vi "emi_Error Filter Array.vi"(1 "Action(No Error)":T2, 5 "Error Codes":i32[](array[numeric]), 9 "error in (no error)":errorcluster, 12 "Filter(Error&Warning)":T1) -> (8 "Filter Triggered":bool, 10 "error out":errorcluster)   [LabVIEW 2011]
doc: "Filter error codes based on code(s). \n\nIf Code does not match, no action.\n\nIf code matches, the following is carried out:\nAction = No Error: Remove error.\nAction = Warning: Change from error to warning.\nAction = Error: Leave as Error.\nFilter Triggered is set to True.\n\nIf filtering both Warnings and errors, use bothe Error Filter.vi and Warning Filter.vi"
uses:
  emi_Error&Warning Filter Action.ctl
  _emi_Filter type.ctl
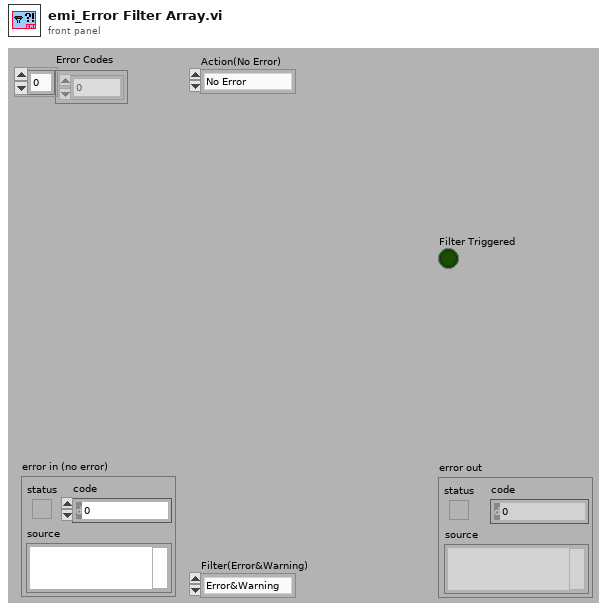
[diagram p1: front panel]
types:
  T1 = typedef "_emi_Filter type.ctl" = enum16{"Error&Warning", "Warning", "Error"}
  T2 = typedef "emi_Error&Warning Filter Action.ctl" = enum16{"No Error", "Warning", "Error"}
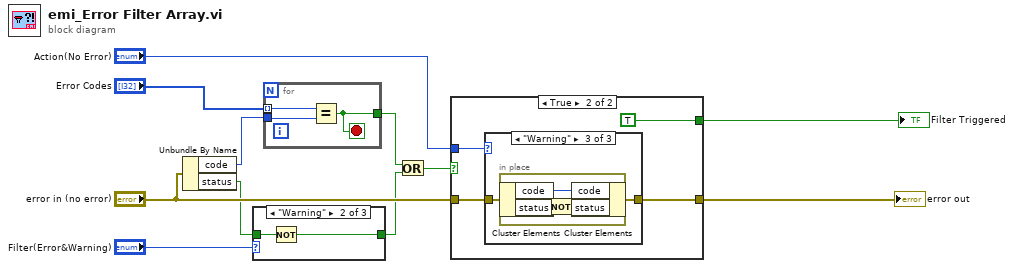
[diagram p0: block diagram]
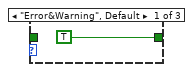
[diagram p2: hidden frame]
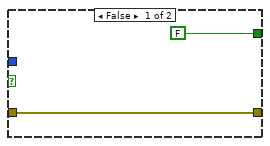
[diagram p4: hidden frame]
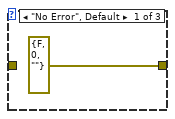
[diagram p5: hidden frame]
diagram:
  n1 = Unbundle By Name("error in (no error)") -> ("code"=w6:i32, "status"=w2:bool)
  n2 = case shown="\"Warning\"" "Filter(Error&Warning)" {
    tunnel: w2 -> [_ w14 w15]
    tunnel: [TRUE w13 w15] -> w1
    frame "Error&Warning", Default {
    }
    frame "Warning" {
      n3 = Not(x=w14) -> (.not. x?=w13:bool)
    }
    frame "Error" {
    }
  }
  n4 = for {
    tunnel: "Error Codes" -> [w18] mode=indexing
    tunnel: w6 -> [w17]
    tunnel: [w16] -> w5
    stop <- w16 stop-if-true
    n5 = Equal?(x=w18, y=w17) -> (x = y?=w16:bool)
  }
  n6 = Or(x=w5, y=w1) -> (x .or. y?=w4:bool)
  n7 = case shown="True" w4 {
    tunnel: [w20 w24] -> w10
    tunnel: "error in (no error)" -> [w20 w23]
    tunnel: "Action(No Error)" -> [_ w22]
    tunnel: [FALSE TRUE] -> w7
    frame False {
    }
    frame True {
      n8 = case shown="\"Warning\"" w22 {
        tunnel: [errorcluster {"status"=FALSE, "code"=0, "source"=""} ("error IO") w26 w27] -> w24
        tunnel: w23 -> [_ w26 w28]
        frame "No Error", Default {
        }
        frame "Error" {
        }
        frame "Warning" {
          n9 = in-place {
            n10 = in-place-cluster #1(w28) -> ("code"=w31:i32, "status"=w29:bool)
            n11 = Not(x=w29) -> (.not. x?=w30:bool)
            n12 = in-place-cluster #1("code"=w31, "status"=w30) -> (w27:errorcluster)
          }
        }
      }
    }
  }
  "error out" <- w10
  "Filter Triggered" <- w7
